vi "SpectrometerTest.vi"() -> ()   [LabVIEW 2015]
uses:
  <vilib>/Utility/file.llb/Write Delimited Spreadsheet (DBL).vi
panel:
  out "存储路径 2":path
  in  "暗噪声采集":bool
  out "存储路径":path
  out "Spectrum of the first Spectrometer":cluster{"Y":dbl[], "Y":dbl[]}[](graph)
  in  "stop":bool
  in  "Enter the \nInetegration Time":i32=100000
  in  "Start":bool
  out "Number of Spectrometers":i32
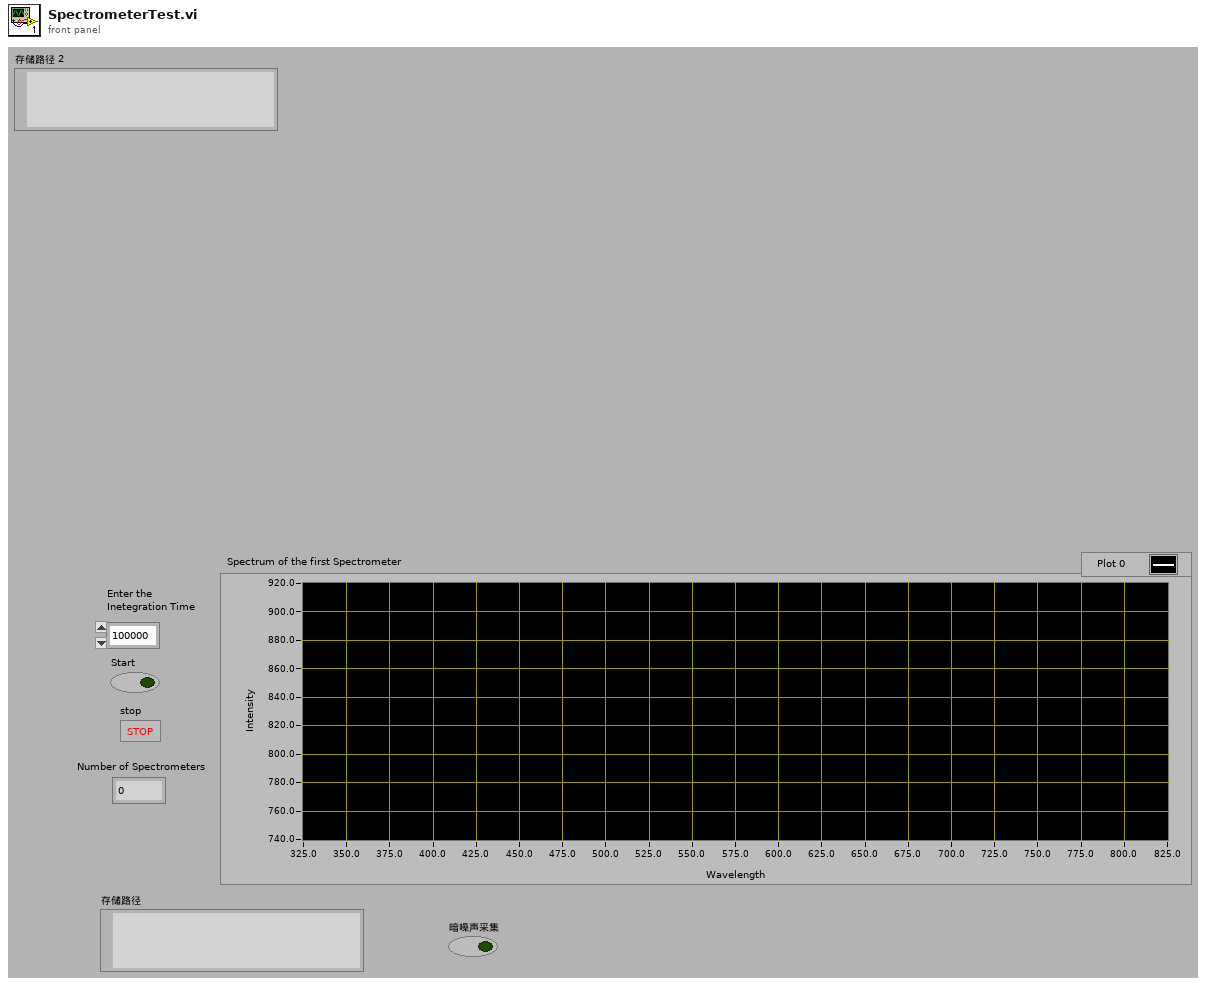
[diagram p1: front panel]
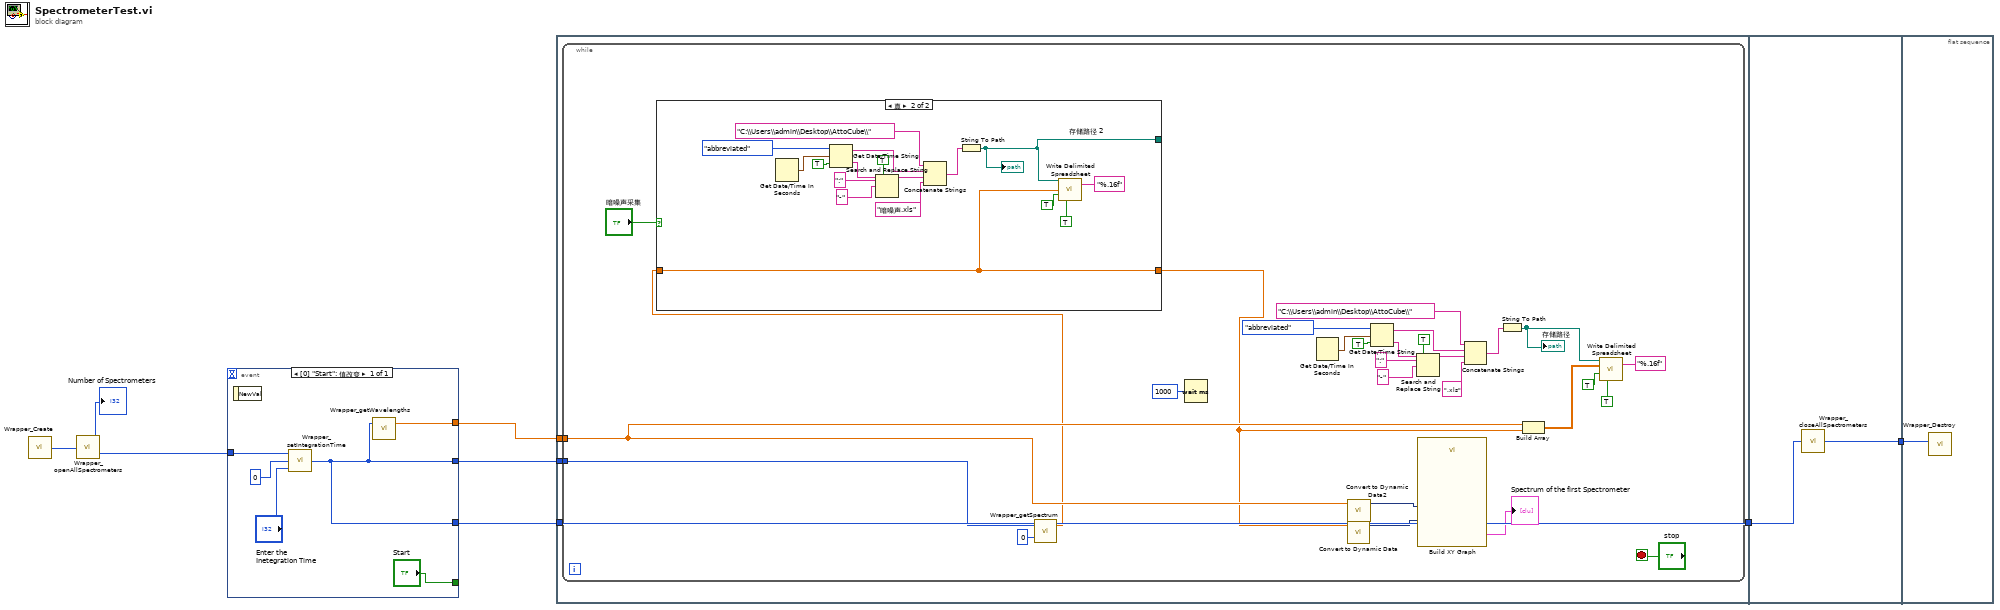
[diagram p0: block diagram]
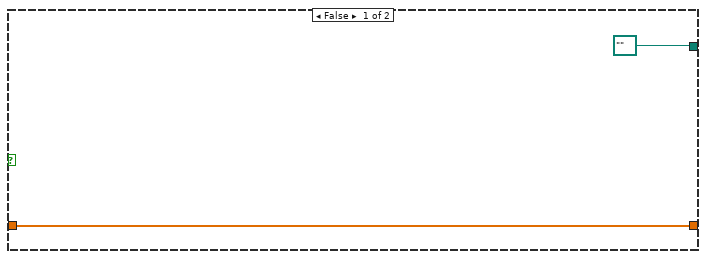
[diagram p2: hidden frame]
diagram:
  n1 = call <userlib>:"Wrapper_Create.vi"() -> ("Wrapper"=w8:u32)
  n2 = call <userlib>:"Wrapper_openAllSpectrometers.vi"("Wrapper In"=w8) -> ("Number of Spectrometers"=→"Number of Spectrometers":i32, "Wrapper Out"=w6:u32)
  n3 = event shown="[0] \"Start\": 值改变" {
    selector: _ -> [_]
    dyn-events: _ -> [_]
    timeout: _ -> [_]
    tunnel: ["Start"] -> _
    tunnel: w6 -> [w11]
    tunnel: [w9] -> w5
    tunnel: [w10] -> w4
    tunnel: [w9] -> w2
    event "Start": Value Change {
      n4 = event-data() -> ()  [unwired: 1 in, 1 out]
      n5 = call <userlib>:"Wrapper_setIntegrationTime.vi"("Integration Time"="Enter the \nInetegration Time", "Index"=0, "Wrapper In"=w11) -> ("Wrapper Out"=w9:u32)
      n6 = call <userlib>:"Wrapper_getWavelengths.vi"("Wrapper"=w9) -> ("WL Values"=w10:dbl[])  [unwired: 1 in, 1 out]
    }
  }
  n7 = flat-sequence {
    tunnel: w5 -> [w17]
    tunnel: w4 -> [w16]
    tunnel: [w15] -> w3
    tunnel: w2 -> [w15]
    tunnel: w3 -> [w66]
    tunnel: [w65] -> w1
    tunnel: w1 -> [w67]
    frame #0 {
      n8 = while {
        tunnel: w17 -> [w45]
        tunnel: w16 -> [w20]
        stop <- "stop" stop-if-true
        n9 = call <userlib>:"Wrapper_getSpectrum.vi"("Index"=0, "Wrapper"=w45) -> ("Spectrum Values"=w19:dbl[])  [unwired: 1 out]
        n10 = case shown="真" "暗噪声采集" {
          tunnel: w19 -> [w47 w49]
          tunnel: [w47 w49] -> w18
          tunnel: [path "" w48] -> _
          frame False {
          }
          frame True {
            n11 = Get Date/Time In Seconds() -> (seconds since 1Jan1904=w64:timestamp)
            n12 = Get Date/Time String(date format (0)=enum16{"short", "long", "abbreviated"}."abbreviated" ("日期格式(0)"), seconds (now)=w64, want seconds? (F)=TRUE ("需要秒？(F)")) -> (date string=w56:string, time string=w61:string)
            n13 = Search and Replace String(replace all?=TRUE ("替换全部？(F)"), input string=w61, search string=":" ("搜索字符串"), replace string="-" ("替换字符串(\"\")")) -> (result string=w57:string)  [unwired: 4 in, 3 out]
            n14 = Concatenate Strings("C:\\Users\\admin\\Desktop\\AttoCube\\" ("字符串"), w56, w57, "暗噪声.xls" ("字符串")) -> (w55:string)
            n15 = String To Path(string=w55) -> (path=w48:path)
            "存储路径 2" <- w48
            n16 = call-poly <vilib>:"Write Delimited Spreadsheet.vi"("file path (dialog if empty)"=w48, "format (%.3f)"="%.16f", "1D data"=w49, "append to file? (F)"=TRUE, "transpose? (F)"=TRUE) -> ()  [unwired: 9 in, 2 out]
          }
        }
        n17 = Wait (ms)(milliseconds to wait=u32 1000 ("等待时间（毫秒）")) -> ()  [unwired: 1 out]
        n18 = Get Date/Time In Seconds() -> (seconds since 1Jan1904=w41:timestamp)
        n19 = call "Convert to Dynamic Data"("Array"=w18) -> ("Dynamic Data Type"=w24:dynamicdata)  [unwired: 3 in]
        n20 = call "Convert to Dynamic Data2"("Array"=w20) -> ("Dynamic Data Type"=w25:dynamicdata)  [unwired: 3 in]
        n21 = Get Date/Time String(date format (0)=enum16{"short", "long", "abbreviated"}."abbreviated" ("日期格式(0)"), seconds (now)=w41, want seconds? (F)=TRUE ("需要秒？(F)")) -> (date string=w33:string, time string=w38:string)
        n22 = Search and Replace String(replace all?=TRUE ("替换全部？(F)"), input string=w38, search string=":" ("搜索字符串"), replace string="-" ("替换字符串(\"\")")) -> (result string=w34:string)  [unwired: 4 in, 3 out]
        n23 = call "Build XY Graph"("Y Input"=w24, "X Input"=w25) -> ("XY Graph"=→"Spectrum of the first Spectrometer":cluster{"Y":dbl[], "Y":dbl[]}[])  [unwired: 8 in, 1 out]
        n24 = Concatenate Strings("C:\\Users\\admin\\Desktop\\AttoCube\\" ("字符串"), w33, w34, ".xls" ("字符串")) -> (w32:string)
        n25 = String To Path(string=w32) -> (path=w29:path)
        "存储路径" <- w29
        n26 = Build Array(w20, w18) -> (w23:dbl[][])
        n27 = call-poly <vilib>:"Write Delimited Spreadsheet.vi"("file path (dialog if empty)"=w29, "format (%.3f)"="%.16f", "2D data"=w23, "append to file? (F)"=TRUE, "transpose? (F)"=TRUE) -> ()  [unwired: 9 in, 2 out]
      }
    }
    frame #1 {
      n28 = call <userlib>:"Wrapper_closeAllSpectrometers.vi"("Wrapper In"=w66) -> ("Wrapper Out"=w65:u32)
    }
    frame #2 {
      n29 = call <userlib>:"Wrapper_Destroy.vi"("Wrapper"=w67) -> ()
    }
  }
